vi "get image.vi"(7 "Image Logging Prefix":string="Image", 8 "error in":errorcluster, 9 "Image Logging Path":path=path "c:/", 10 "Log Image":bool=TRUE, 11 "Stop (F)":bool) -> (0 "error out":errorcluster, 1 "Image Number":u32, 2 "Frame Rate":dbl, 3 "Image Out":T1(plugin-control), 4 "Stopped":bool)   [LabVIEW 2015]
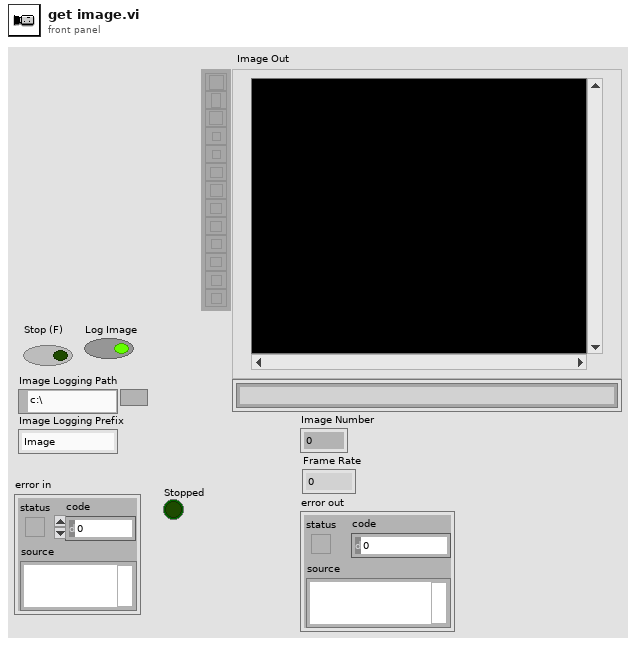
[diagram p1: front panel]
types:
  T1 = typedef "IMAQ Image.ctl" = refnum<image>
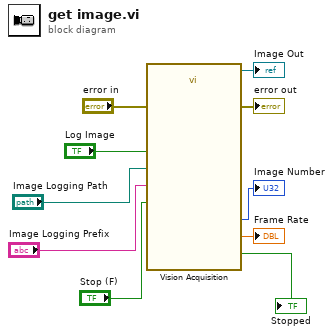
[diagram p0: block diagram]
diagram:
  n1 = call "Vision Acquisition"("Log Image"="Log Image", "Image Logging Path"="Image Logging Path", "Image Logging Prefix"="Image Logging Prefix", "Stop (F)"="Stop (F)", "error in"="error in") -> ("Image Out"=→"Image Out":T1, "Image Number"=→"Image Number":u32, "Frame Rate"=→"Frame Rate":dbl, "Stopped"=→"Stopped":bool, "error out"=→"error out":errorcluster)  [unwired: 18 in]
